vi "Digital Clock.vi"() -> ()   [LabVIEW 2011]
panel:
  out "Shi wei shu of Sec":dbl
  out "Ge wei shu of Sec":dbl
  out "Shi wei shu of Hour":dbl
  out "Ge wei shu of Hour":dbl
  out "Shi wei shu of Min":dbl
  out "Ge wei shu of Min":dbl
  out "Hour":dbl
  out "Second":dbl
  out "Minute":dbl
  in  "stop":bool
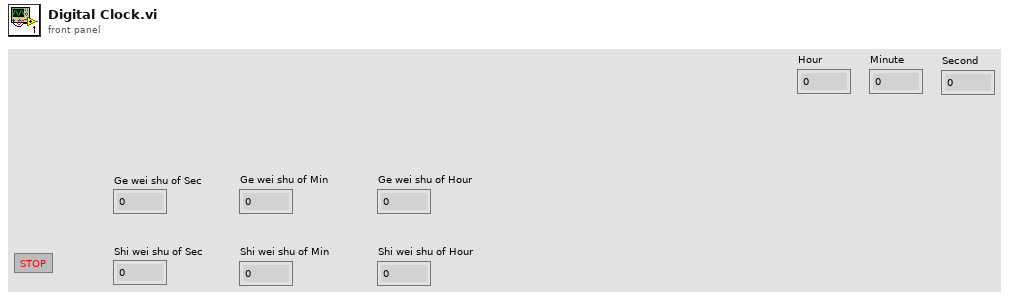
[diagram p1: front panel]
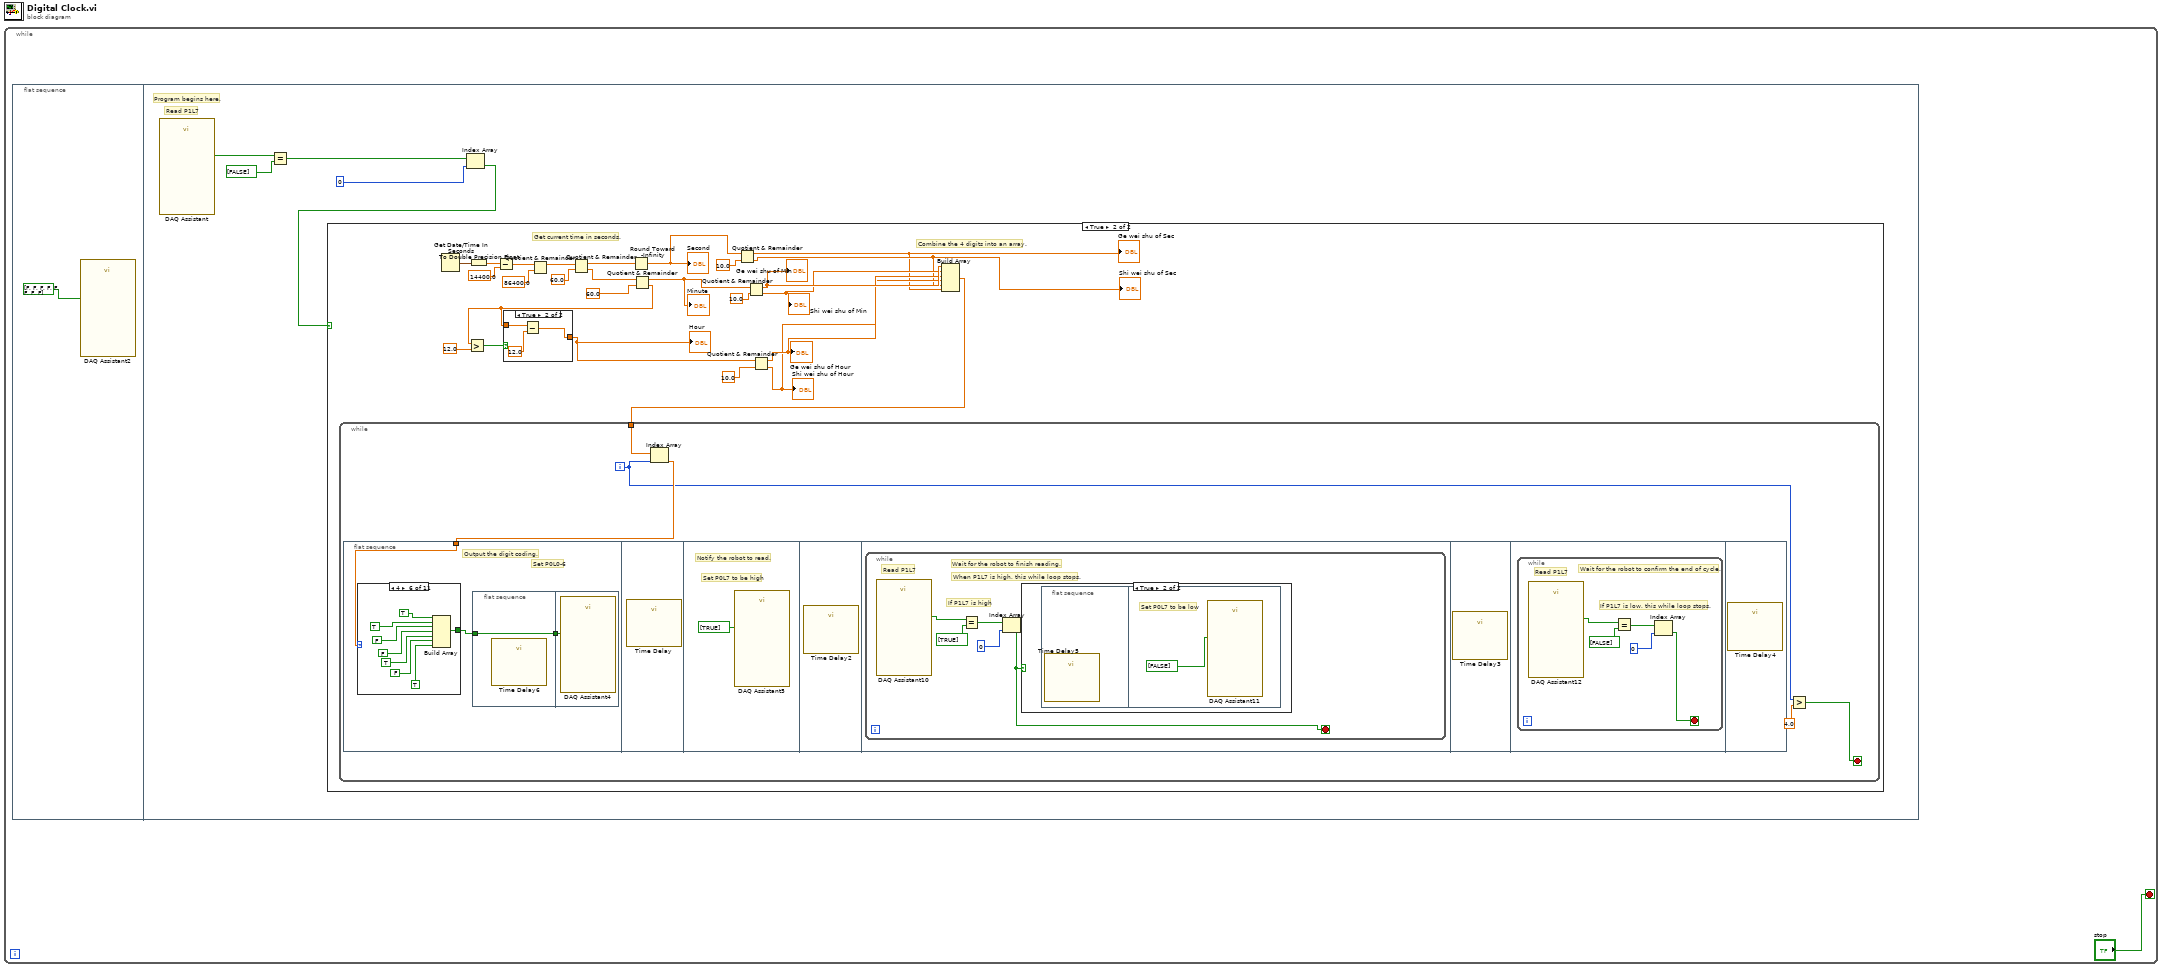
[diagram p0: block diagram]
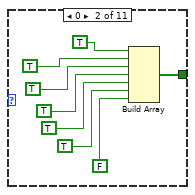
[diagram p4: hidden frame]
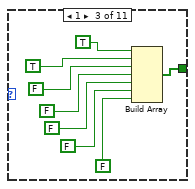
[diagram p5: hidden frame]
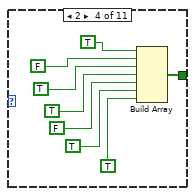
[diagram p6: hidden frame]
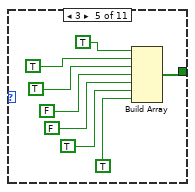
[diagram p7: hidden frame]
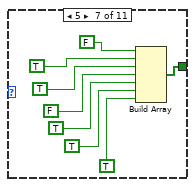
[diagram p8: hidden frame]
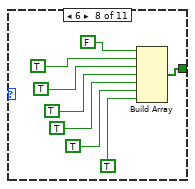
[diagram p9: hidden frame]
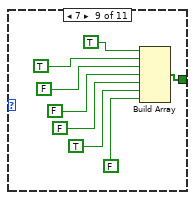
[diagram p10: hidden frame]
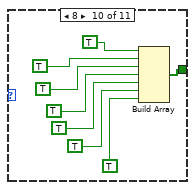
[diagram p11: hidden frame]
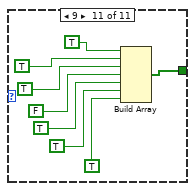
[diagram p12: hidden frame]
diagram:
  n1 = while {
    stop <- "stop" stop-if-true
    n2 = flat-sequence {
      frame #0 {
        n3 = call "DAQ Assistant2"("data"=bool[] [FALSE, FALSE, FALSE, FALSE, FALSE, FALSE, FALSE, FALSE]) -> ()  [unwired: 17 in, 2 out]
      }
      frame #1 {
        # "Program begins here."
        # "Read P1L7"
        n4 = call "DAQ Assistant"() -> ("data"=w7:bool[])  [unwired: 17 in, 2 out]
        n5 = Equal?(x=w7, y=bool[] [FALSE]) -> (x = y?=w5:bool[])
        n6 = Index Array(array=w5, index=0) -> (element=w3:bool)
        n7 = case shown="True" w3 {
          frame False {
          }
          frame True {
            # "Combine the 4 digits into an array."
            # "Get current time in seconds."
            n8 = Get Date/Time In Seconds() -> (seconds since 1Jan1904=w17:timestamp)
            n9 = To Double Precision Float(number=w17) -> (double precision float=w26:dbl)
            n10 = Subtract(x=w26, y=14400.0) -> (x-y=w28:dbl)
            n11 = Quotient & Remainder(x=w28, y=86400.0) -> (x-y*floor(x/y)=w19:dbl)  [unwired: 1 out]
            n12 = Quotient & Remainder(x=w19, y=60.0) -> (x-y*floor(x/y)=w23:dbl, floor(x/y)=w21:dbl)
            n13 = Round Toward -Infinity(1:w23) -> (0:w15:dbl)
            "Second" <- w15
            n14 = Quotient & Remainder(x=w21, y=60.0) -> (x-y*floor(x/y)=w30:dbl, floor(x/y)=w29:dbl)
            "Minute" <- w30
            n15 = Greater?(x=w29, y=12.0) -> (0:w24:bool)
            n16 = case shown="True" w24 {
              tunnel: w29 -> [w136 w139]
              tunnel: [w136 w137] -> w32
              frame False {
              }
              frame True {
                n17 = Subtract(x=w139, y=12.0) -> (x-y=w137:dbl)
              }
            }
            "Hour" <- w32
            n18 = Quotient & Remainder(x=w15, y=10.0) -> (x-y*floor(x/y)=w8:dbl, floor(x/y)=w9:dbl)
            "Ge wei shu of Sec" <- w8
            "Shi wei shu of Sec" <- w9
            n19 = Quotient & Remainder(x=w30, y=10.0) -> (x-y*floor(x/y)=w13:dbl, floor(x/y)=w12:dbl)
            "Ge wei shu of Min" <- w13
            "Shi wei shu of Min" <- w12
            n20 = Quotient & Remainder(x=w32, y=10.0) -> (x-y*floor(x/y)=w11:dbl, floor(x/y)=w10:dbl)
            "Ge wei shu of Hour" <- w11
            "Shi wei shu of Hour" <- w10
            n21 = Build Array(w13, w12, w11, w10, w9, w8) -> (w16:dbl[])
            n22 = while {
              tunnel: w16 -> [w38]
              i -> [w35]
              stop <- w34 stop-if-true
              n23 = flat-sequence {
                tunnel: w37 -> [w39]
                frame #0 {
                  # "Output the digit coding."
                  # "Set P0L0-6"
                  n24 = case shown="4" w39 {
                    tunnel: [_ w44 w52 w60 w68 w76 w84 w92 w100 w108 w116] -> w41
                    frame Default {
                    }
                    frame 0 {
                      n25 = Build Array(TRUE, TRUE, TRUE, TRUE, TRUE, TRUE, FALSE) -> (w44:bool[])
                    }
                    frame 1 {
                      n26 = Build Array(TRUE, TRUE, FALSE, FALSE, FALSE, FALSE, FALSE) -> (w52:bool[])
                    }
                    frame 2 {
                      n27 = Build Array(TRUE, FALSE, TRUE, TRUE, FALSE, TRUE, TRUE) -> (w60:bool[])
                    }
                    frame 3 {
                      n28 = Build Array(TRUE, TRUE, TRUE, FALSE, FALSE, TRUE, TRUE) -> (w68:bool[])
                    }
                    frame 4 {
                      n29 = Build Array(TRUE, TRUE, FALSE, FALSE, TRUE, FALSE, TRUE) -> (w76:bool[])
                    }
                    frame 5 {
                      n30 = Build Array(FALSE, TRUE, TRUE, FALSE, TRUE, TRUE, TRUE) -> (w84:bool[])
                    }
                    frame 6 {
                      n31 = Build Array(FALSE, TRUE, TRUE, TRUE, TRUE, TRUE, TRUE) -> (w92:bool[])
                    }
                    frame 7 {
                      n32 = Build Array(TRUE, TRUE, FALSE, FALSE, FALSE, TRUE, FALSE) -> (w100:bool[])
                    }
                    frame 8 {
                      n33 = Build Array(TRUE, TRUE, TRUE, TRUE, TRUE, TRUE, TRUE) -> (w108:bool[])
                    }
                    frame 9 {
                      n34 = Build Array(TRUE, TRUE, TRUE, FALSE, TRUE, TRUE, TRUE) -> (w116:bool[])
                    }
                  }
                  n35 = flat-sequence {
                    tunnel: w41 -> [w42]
                    tunnel: [w42] -> w40
                    tunnel: w40 -> [w43]
                    frame #0 {
                      n36 = call "Time Delay6"() -> ()  [unwired: 11 in, 1 out]
                    }
                    frame #1 {
                      n37 = call "DAQ Assistant4"("data"=w43) -> ()  [unwired: 17 in, 2 out]
                    }
                  }
                }
                frame #1 {
                  n38 = call "Time Delay"() -> ()  [unwired: 11 in, 1 out]
                }
                frame #2 {
                  # "Notify the robot to read."
                  # "Set P0L7 to be high"
                  n39 = call "DAQ Assistant5"("data"=bool[] [TRUE]) -> ()  [unwired: 17 in, 2 out]
                }
                frame #3 {
                  n40 = call "Time Delay2"() -> ()  [unwired: 11 in, 1 out]
                }
                frame #4 {
                  n41 = while {
                    stop <- w125 stop-if-true
                    # "Wait for the robot to finish reading."
                    # "When P1L7 is high, this while loop stops."
                    # "If P1L7 is high"
                    # "Read P1L7"
                    n42 = call "DAQ Assistant10"() -> ("data"=w129:bool[])  [unwired: 17 in, 2 out]
                    n43 = Equal?(x=w129, y=bool[] [TRUE]) -> (x = y?=w126:bool[])
                    n44 = Index Array(array=w126, index=0) -> (element=w125:bool)
                    n45 = case shown="True" w125 {
                      frame False {
                      }
                      frame True {
                        n46 = flat-sequence {
                          frame #0 {
                            n47 = call "Time Delay5"() -> ()  [unwired: 11 in, 1 out]
                          }
                          frame #1 {
                            # "Set P0L7 to be low"
                            n48 = call "DAQ Assistant11"("data"=bool[] [FALSE]) -> ()  [unwired: 17 in, 2 out]
                          }
                        }
                      }
                    }
                  }
                }
                frame #5 {
                  n49 = call "Time Delay3"() -> ()  [unwired: 11 in, 1 out]
                }
                frame #6 {
                  n50 = while {
                    stop <- w131 stop-if-true
                    # "Wait for the robot to confirm the end of cycle."
                    # "If P1L7 is low, this while loop stops."
                    # "Read P1L7"
                    n51 = call "DAQ Assistant12"() -> ("data"=w135:bool[])  [unwired: 17 in, 2 out]
                    n52 = Equal?(x=w135, y=bool[] [FALSE]) -> (x = y?=w132:bool[])
                    n53 = Index Array(array=w132, index=0) -> (element=w131:bool)
                  }
                }
                frame #7 {
                  n54 = call "Time Delay4"() -> ()  [unwired: 11 in, 1 out]
                }
              }
              n55 = Index Array(array=w38, index=w35) -> (element=w37:dbl)
              n56 = Greater?(x=w35, y=4.0) -> (0:w34:bool)
            }
          }
        }
      }
    }
  }
